vi "(SubVI) Write to Three AxisesPI_YCC.vi"(4 "Position wrote to three axis (um)":dbl) -> ()   [LabVIEW 2014]
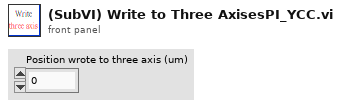
[diagram p1: front panel]
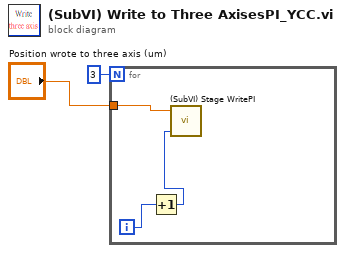
[diagram p0: block diagram]
diagram:
  n1 = for {
    N: 3 -> [_]
    tunnel: "Position wrote to three axis (um)" -> [w3]
    i -> [w5]
    n2 = Increment(x=w5) -> (x+1=w4:i32)
    n3 = call "(SubVI) Stage WritePI.vi"("axis"=w4, "position"=w3) -> ()  [unwired: 4 in]
  }
